vi "GetElementBG.vi"(6 "error in":errorcluster, 9 "Array in":refnum<class "Array.lvclass">) -> (0 "error out":errorcluster, 3 "Array out":refnum<class "Array.lvclass">, 4 "Element BG":u32(colorbox))   [LabVIEW 2014, in "Array.lvclass"]
uses:
  Array.lvclass
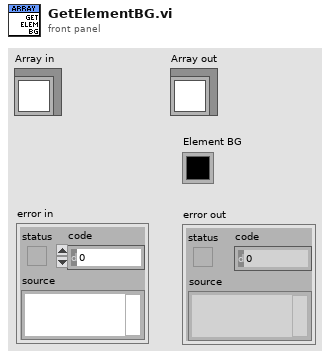
[diagram p1: front panel]
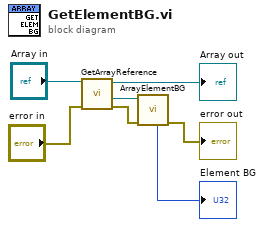
[diagram p0: block diagram]
diagram:
  n1 = call "GetArrayReference.vi"("error in"="error in", "Array in"="Array in") -> ("error out"=w4:errorcluster, "array reference"=w5:refnum<vi>, "Array out"=→"Array out":refnum<class "Array.lvclass">)  [unwired: 7 in]
  n2 = call "ArrayElementBG.vi"("error in"=w4, "Arr Refnum"=w5) -> ("error out"=→"error out":errorcluster, "Element BG"=→"Element BG":u32)  [unwired: 7 in, 1 out]
